vi "Close.vi"(8 "error in (no error)":errorcluster, 11 "queue out":refnum<queue>) -> (0 "error out":errorcluster)   [LabVIEW 2019, in "Simple Queue Message.lvlib"]
uses:
  Simple Queue Message.lvlib
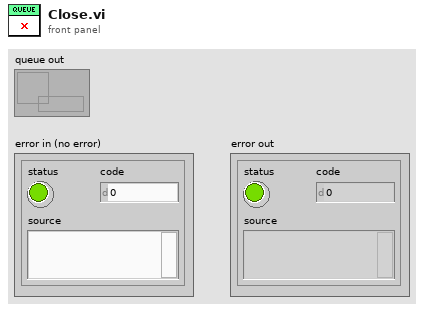
[diagram p1: front panel]
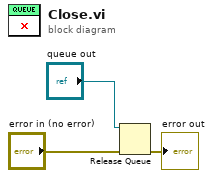
[diagram p0: block diagram]
diagram:
  n1 = Release Queue(queue="queue out", error in (no error)="error in (no error)") -> (error out=→"error out":errorcluster)  [unwired: 1 in, 2 out]
